vi "Error Converter (ErrCode or Status).vi"(8 "error in (no error)":errorcluster, 11 "error code":i32) -> (0 "error out":errorcluster)   [LabVIEW 2011, in "libPhyspec.lvlib"]
uses:
  libPhyspec.lvlib
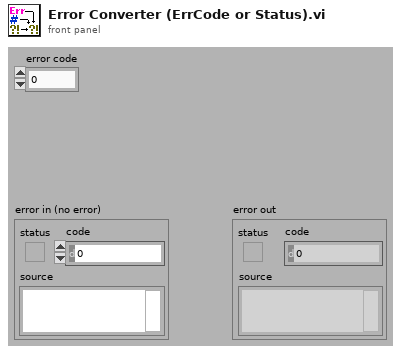
[diagram p1: front panel]
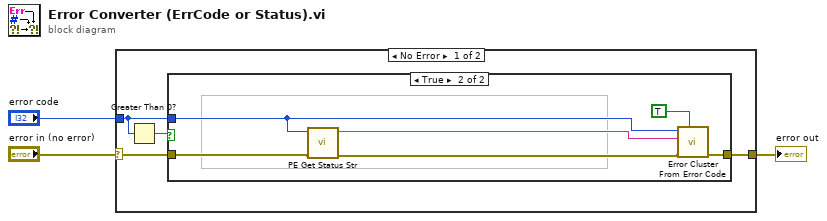
[diagram p0: block diagram]
diagram:
  n1 = case shown="No Error" "error in (no error)" {
    selector: "error in (no error)" -> [w7 w15]
    tunnel: [w6 w15] -> w2
    tunnel: "error code" -> [w4 _]
    frame No Error {
      n2 = Greater Than 0?(x=w4) -> (x > 0?=w5:bool)
      n3 = case shown="True" w5 {
        tunnel: w7 -> [w8 w12]
        tunnel: w4 -> [_ w10]
        tunnel: [w8 w14] -> w6
        frame False {
        }
        frame True {
          n4 = call "PE Get Status Str.vi"("error in (no error)"=w12, "code"=w10) -> ("error out"=w11:errorcluster, "function return"=w9:string)  [unwired: 8 in]
          n5 = call <vilib>:"Error Cluster From Error Code.vi"("show call chain? (False)"=TRUE, "error in (no error)"=w11, "error message (\"\")"=w9, "error code (0)"=w10) -> ("error out"=w14:errorcluster)  [unwired: 5 in]
        }
      }
    }
    frame Error {
    }
  }
  "error out" <- w2
